vi "Configuration parameter reading.vi"(8 "error in (no error)":errorcluster caption="错误输入（无错误）") -> (0 "error out":errorcluster caption="错误输出", 1 "串口打开":bool, 2 "baud rate (9600)":u32(ring)=19200 caption="波特率" items=["1200"=1200, "2400"=2400, "4800"=4800, "9600"=9600, "19200"=19200, "38400"=38400, "115200"=115200], 3 "VISA resource name":refnum<visa-resource-name> caption="串口", 5 "运行模式":enum16{"维护模式", "常规模式"}(ring)=enum."常规模式")   [LabVIEW 2016, in "流量计集成.lvlib" / "SL1500-3G.lvlib"]
uses:
  SL1500-3G.lvlib
  <vilib>/Utility/config.llb/Read Key (String).vi
  <vilib>/Utility/config.llb/Read Key (U32).vi
  <vilib>/Utility/config.llb/Read Key (I32).vi
  <vilib>/Utility/config.llb/Read Key (Boolean).vi
  <vilib>/Utility/config.llb/NI_LVConfig.lvlib
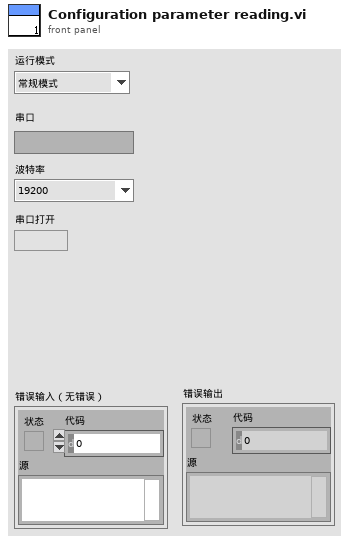
[diagram p1: front panel]
types:
  T1 = typedef "NI_LVConfig.lvlib/Config Data RefNum.ctl" = refnum<k1>
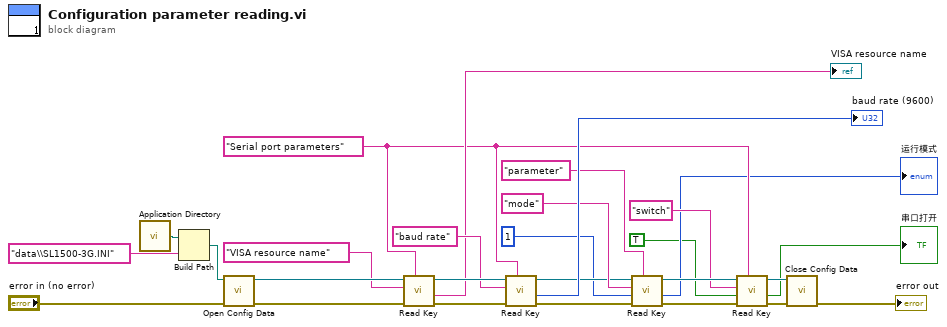
[diagram p0: block diagram]
diagram:
  w5 = "Serial port parameters" ("section")
  n1 = call <vilib>:"Application Directory.vi"() -> ("Application Directory"=w24:path)
  n2 = Build Path(base path=w24, name or relative path="data\\SL1500-3G.INI" ("名称或相对路径")) -> (appended path=w25:path)
  n3 = call <vilib>:"Open Config Data.vi"("error in (no error)"="error in (no error)", "configuration file path"=w25) -> ("error out"=w26:errorcluster, "refnum"=w27:T1)  [unwired: 7 in, 1 out]
  n4 = call-poly <vilib>:"Read Key.vi"("section"=w5, "error in (no error)"=w26, "key"="VISA resource name", "refnum"=w27) -> ("error out"=w20:errorcluster, "value"=→"VISA resource name":string, "refnum out"=w21:T1)  [unwired: 4 in, 1 out]
  n5 = call-poly <vilib>:"Read Key.vi"("section"=w5, "error in (no error)"=w20, "key"="baud rate", "refnum"=w21) -> ("error out"=w8:errorcluster, "value"=→"baud rate (9600)":u32, "refnum out"=w9:T1)  [unwired: 4 in, 1 out]
  n6 = call-poly <vilib>:"Read Key.vi"("section"="parameter", "error in (no error)"=w8, "default value"=1, "key"="mode", "refnum"=w9) -> ("error out"=w13:errorcluster, "value"=→"运行模式":i32, "refnum out"=w14:T1)  [unwired: 3 in, 1 out]
  n7 = call-poly <vilib>:"Read Key.vi"("section"=w5, "error in (no error)"=w13, "default value"=TRUE, "key"="switch", "refnum"=w14) -> ("error out"=w6:errorcluster, "value"=→"串口打开":bool, "refnum out"=w7:T1)  [unwired: 3 in, 1 out]
  n8 = call <vilib>:"Close Config Data.vi"("error in (no error)"=w6, "refnum"=w7) -> ("error out"=→"error out":errorcluster)  [unwired: 8 in, 1 out]
